vi "點檢.vi"() -> ()   [LabVIEW 2015]
uses:
  <vilib>/Utility/miscctls.llb/LVPointTypeDef.ctl
  <vilib>/userdefined/High Color/IMAQdx.ctl
panel:
  out "output cluster":T1
  in  "?":T2={"掃描速度"=1000, "功率"=80, "切割刀數"=10, "角度"=10.0, "掃描速度2"=1000, "功率2"=80, "切割刀數2"=10, "角度2"=10.0, "掃描速度3"=1000, "功率3"=80, "切割刀數3"=10, "角度3"=10.0, "掃描速度4"=1000, "功率4"=80, "切割刀數4"=10, "角度4"=10.0, "掃描速度5"=1000, "功率5"=80, "切割刀數5"=10, "左/右"=""} {"切割刀數5" min=0 max=10 step=1; "功率5" min=3 max=80 step=1; "掃描速度5" min=0 max=10000 step=10; "角度4" min=0.0 max=10.0 step=1.0; "角度3" min=0.0 max=10.0 step=1.0; "角度2" min=0.0 max=10.0 step=1.0; "角度" min=0.0 max=10.0 step=1.0; "切割刀數4" min=0 max=10 step=1; "功率4" min=3 max=80 step=1; "掃描速度4" min=0 max=1000 step=10; "切割刀數3" min=0 max=10 step=1; "功率3" min=3 max=80 step=1; "掃描速度3" min=0 max=1000 step=10; "切割刀數" min=0 max=10 step=1; "功率" min=3 max=80 step=1; "掃描速度" min=0 max=1000 step=10; "切割刀數2" max=10 step=1; "掃描速度2" min=0 max=1000 step=10; "功率2" min=3 max=80 step=1}
  in  "file (use dialog)":path=path "C:/Users/jyun.huang.MINAIK/Desktop/四穴雷切/參數設定/Data/參數設定"
  out "狀態：":string
  out "群組：":string
  out "帳號：":string
  in  "開啟檔案":bool
  in  "儲存檔案":bool
  in  "左/右":enum16{"オ", "右"}(ring)
  in  "雷射半徑":dbl min=0.0 max=220.0
  in  "雷射圓心座標":cluster{"X":dbl, "Y":dbl} {"X" min=0.0 max=220.0}
  in  "雷射觸發":bool
  in  "切割刀數":u32=2 min=2 max=85 step=1
  in  "掃描速率(刀速)":u16=220 max=2000 format="%0.0f"
  in  "功率":u8=70 max=80
  out "前後差異值":cluster{"X差":sgl, "Y差 ":sgl}
  in  "取像":bool
  in  "Tab Control":enum32{"原來圖片                      ", "後來圖片"}(tab)=enum."後來圖片"
  in  "找圓":bool
  in  "差值":bool
  out "原來圓心":cluster{"X ":sgl, "Y":sgl}
  in  "點檢":bool
  out "後來圓心":cluster{"X ":sgl, "Y":sgl}
  out "後來差值":cluster{"X差":sgl, "Y差 ":sgl}
  out "影像中心":cluster{"X":sgl, "Y":sgl}
  out "原來差值":cluster{"X差":sgl, "Y差 ":sgl}
  out "點檢 Action":T3
  out "Image":T4(plugin-control)
  in  "匯入圖片":bool
  in  "離開":bool
  # "每日點檢"
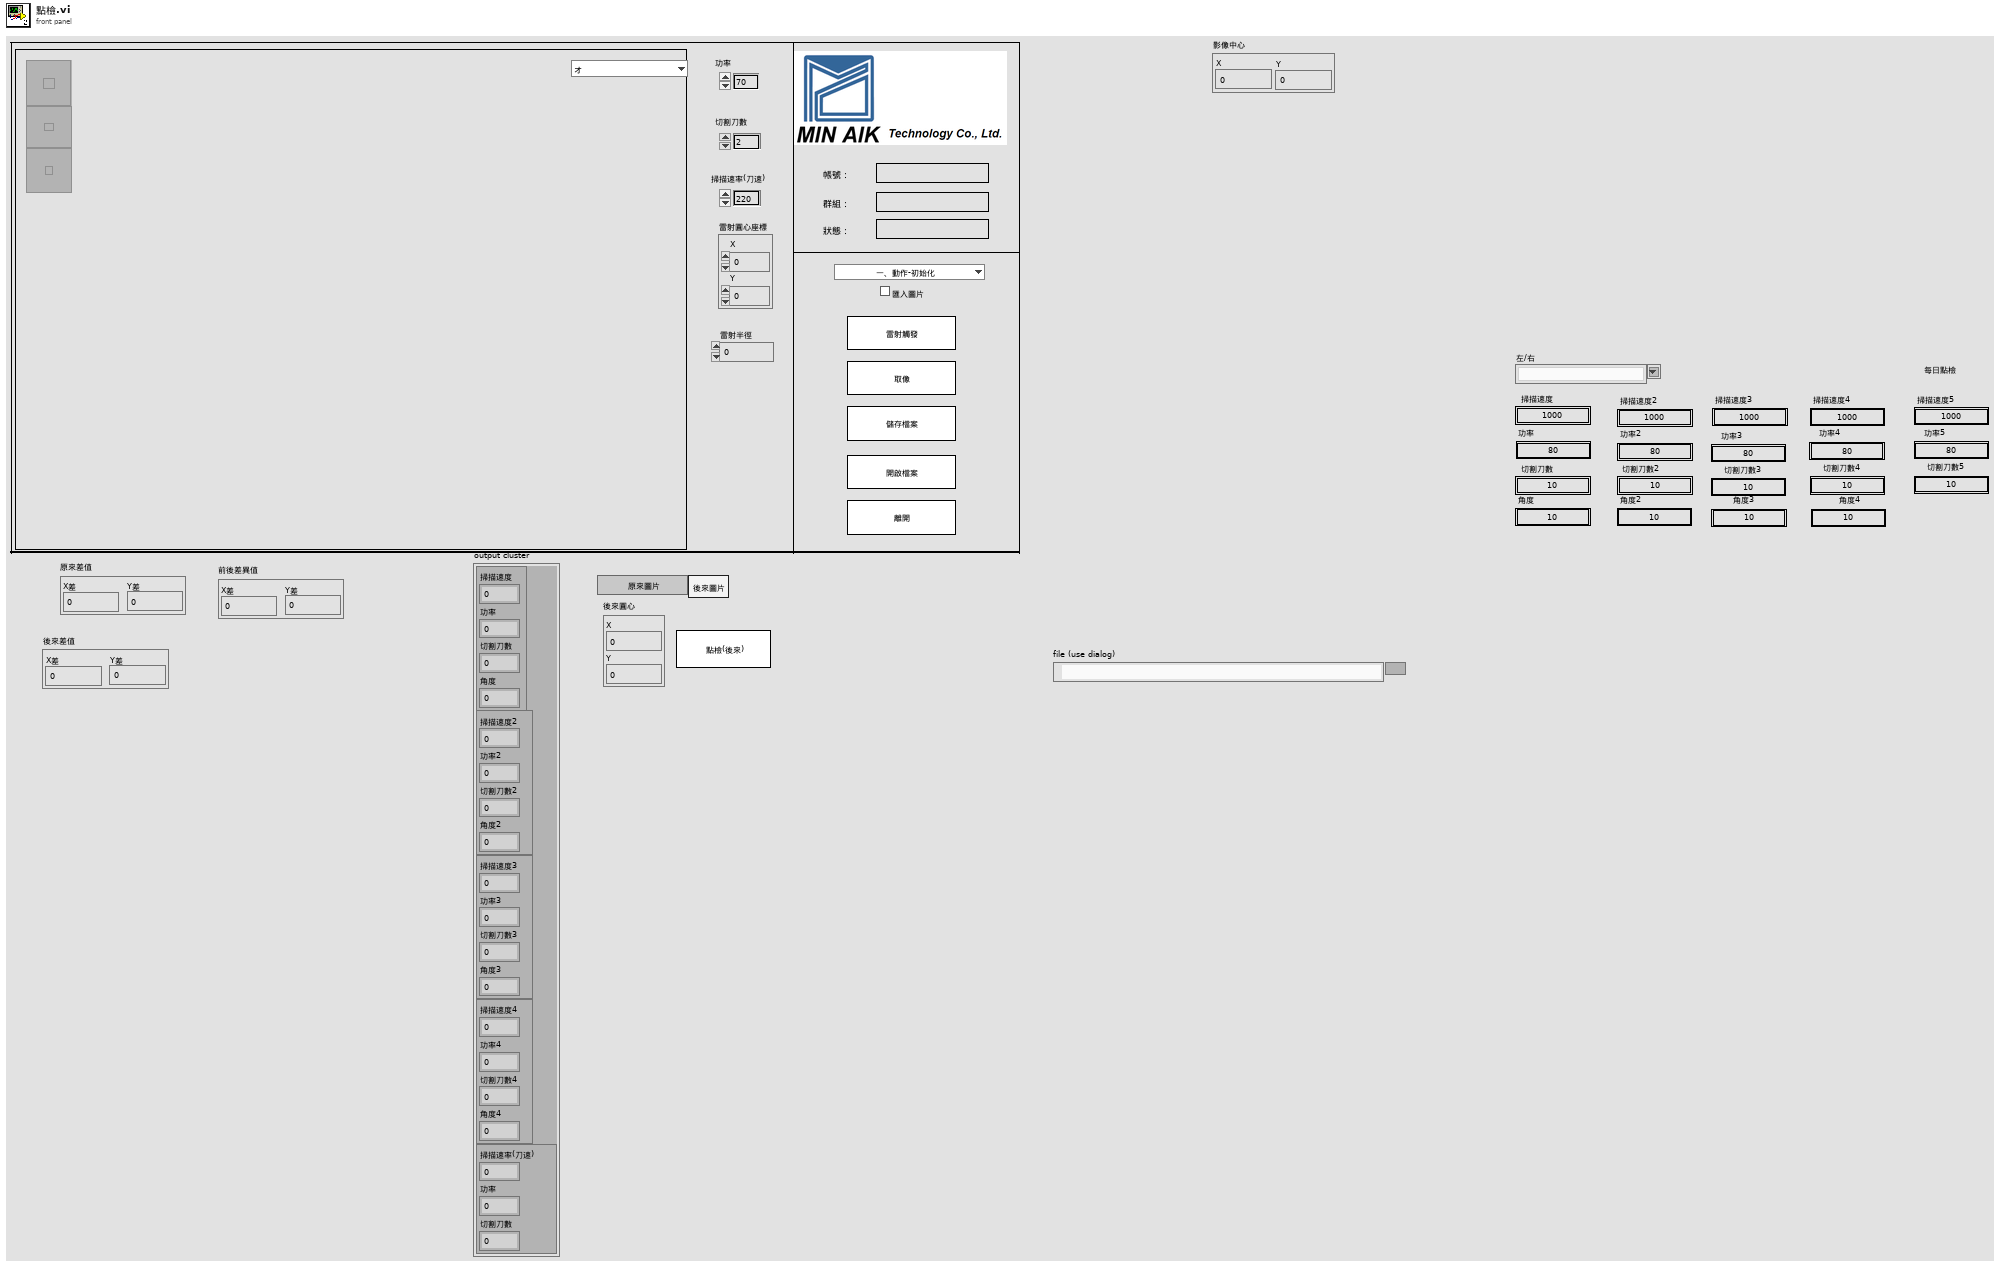
[diagram p1: front panel]
types:
  T1 = cluster{cluster{"掃描速度":i32, "功率":i32, "切割刀數":i32, "角度":dbl}, cluster{"掃描速度2":i32, "功率2":i32, "切割刀數2":i32, "角度2":dbl}, cluster{"掃描速度3":i32, "功率3":i32, "切割刀數3":i32, "角度3":dbl}, cluster{"掃描速度4":i32, "功率4":i32, "切割刀數4":i32, "角度4":dbl}, cluster{"掃描速率(刀速) ":u16, "功率":u8, "切割刀數":u32}}
  T2 = cluster{"掃描速度":i32, "功率":i32, "切割刀數":i32, "角度":dbl, "掃描速度2":i32, "功率2":i32, "切割刀數2":i32, "角度2":dbl, "掃描速度3":i32, "功率3":i32, "切割刀數3":i32, "角度3":dbl, "掃描速度4":i32, "功率4":i32, "切割刀數4":i32, "角度4":dbl, "掃描速度5":i32, "功率5":i32, "切割刀數5":i32, "左/右":string}
  T3 = typedef "點檢_Control_Main Action.ctl" = enum16{"一、動作-初始化", "二、動作-單次取像", "三、動作-測試", "四、動作-點檢", "五、動作-雷射寫入", "六、動作-雷射處發", "七、動作-離開", "1.0 功能-IO控制", "       1.1 IO-初始化", "       1.2 Set Point(EOT On)", "       1.3Set Point(EOT Off)", "       1.4Get Point(SOT)", "2.0功能-相機控制", "       2.1相機-初始化", "       2.2相機-取像", "       2.3相機-關閉", "3.0功能-影像控制", "       3.1影像-初始化", "       3.2影像-更新影像", "       3.3影像-儲存影像", "4.0功能-檢測", "       4.1檢測-初始化", "      4.2檢測-找圓(原來)", "      4.3檢測-找圓(後來)", "5.0功能-雷射控制", "      5.1雷射-初始化", "      5.2雷射-寫入數值", "      5.3雷射-讀出數值", "      5.4雷射-雷射觸發", "      5.5雷射-關閉", "6.0功能-檔案", "       6.1檔案-初始化", "       6.2檔案-儲存檔案", "       6.3檔案-開啟檔案", "       6.4檔案-匯入數值", "7.0 錯誤", "8.0等待", "       8.1等待(計算時間)", "9.0離開", "10.0功能-機台驗證", "      10.1機台驗證-測試", "      10.2機台驗證-檢測", "11.0對話視窗"}
  T4 = typedef "IMAQ Image.ctl" = refnum<image>
  T5 = typedef "LVPointTypeDef.ctl" = cluster{"Horizontal":i16, "Vertical":i16}
  T6 = typedef "IMAQdx.ctl" = refnum<k21>
  T7 = typedef "action_camera.ctl" = enum16{"初始化", "取像", "匯入影像", "結束"}
  T8 = typedef "Image action.ctl" = enum16{"初始化", "創造記憶體", "寫入圖片", "讀取圖片", "刪除圖片", "等待"}
  T9 = typedef "Action_Data.ctl" = enum16{"Initialize", "Get Data", "Set Data", "Delete Data", "Idle"}
  T10 = enum16{"RS232_Init ", "雷射準備訊號", "雷射觸發", "RS232_Close", "寫入雷射XY座標值與角度", "請求程式編號prog所有資訊", "開起導向光", "關閉導向光", "運行切換"}
  T11 = cluster{cluster{"掃描速度":i32, "功率":i32, "切割刀數":dbl, "左/右":string}, cluster{"掃描速度2":i32, "功率2":i32, "切割刀數2":dbl, "左/右":string}, cluster{"掃描速度3":i32, "功率3":i32, "切割刀數3":dbl, "左/右":string}, cluster{"掃描速度4":i32, "功率4":i32, "切割刀數4":dbl, "左/右":string}, cluster{"掃描速度5":i32, "功率5":i32, "切割刀數5":dbl, "左/右":string}}
  T12 = cluster{"功率":u8, "掃描速率(刀速) ":u16, "雷射半徑":dbl, "刀數":u32}
  T13 = cluster{"ROI":cluster{"Global Rectangle":i32[], "Contours":cluster{"Contour Type":u32, "ROI Type":u32, "Points":i32[]}[]}, "圓心 (Pixels)":cluster{"X":sgl, "Y":sgl}}
  T14 = typedef "Image Type" = u32
  T15 = cluster{"Global Rectangle":i32[], "Contours":cluster{"Contour Type":u32, "ROI Type":u32, "Points":i32[]}[]}
  T16 = cluster{"功率":u8, "掃描速率(刀速) ":u16, "雷射半徑":dbl, "切割刀數":u32}
  T17 = cluster{"掃描速度5":i32, "功率5":i32, "切割刀數5":dbl, "左/右":string}
  T18 = cluster{"掃描速度4":i32, "功率4":i32, "切割刀數4":i32, "角度4":dbl}
  T19 = cluster{"掃描速度2":i32, "功率2":i32, "切割刀數2":i32, "角度2":dbl}
  T20 = cluster{"掃描速度3":i32, "功率3":i32, "切割刀數3":i32, "角度3":dbl}
  T21 = cluster{"掃描速度":i32, "功率":i32, "切割刀數":i32, "角度":dbl}
  T22 = cluster{"name or relative path":string, "Variant":variant}
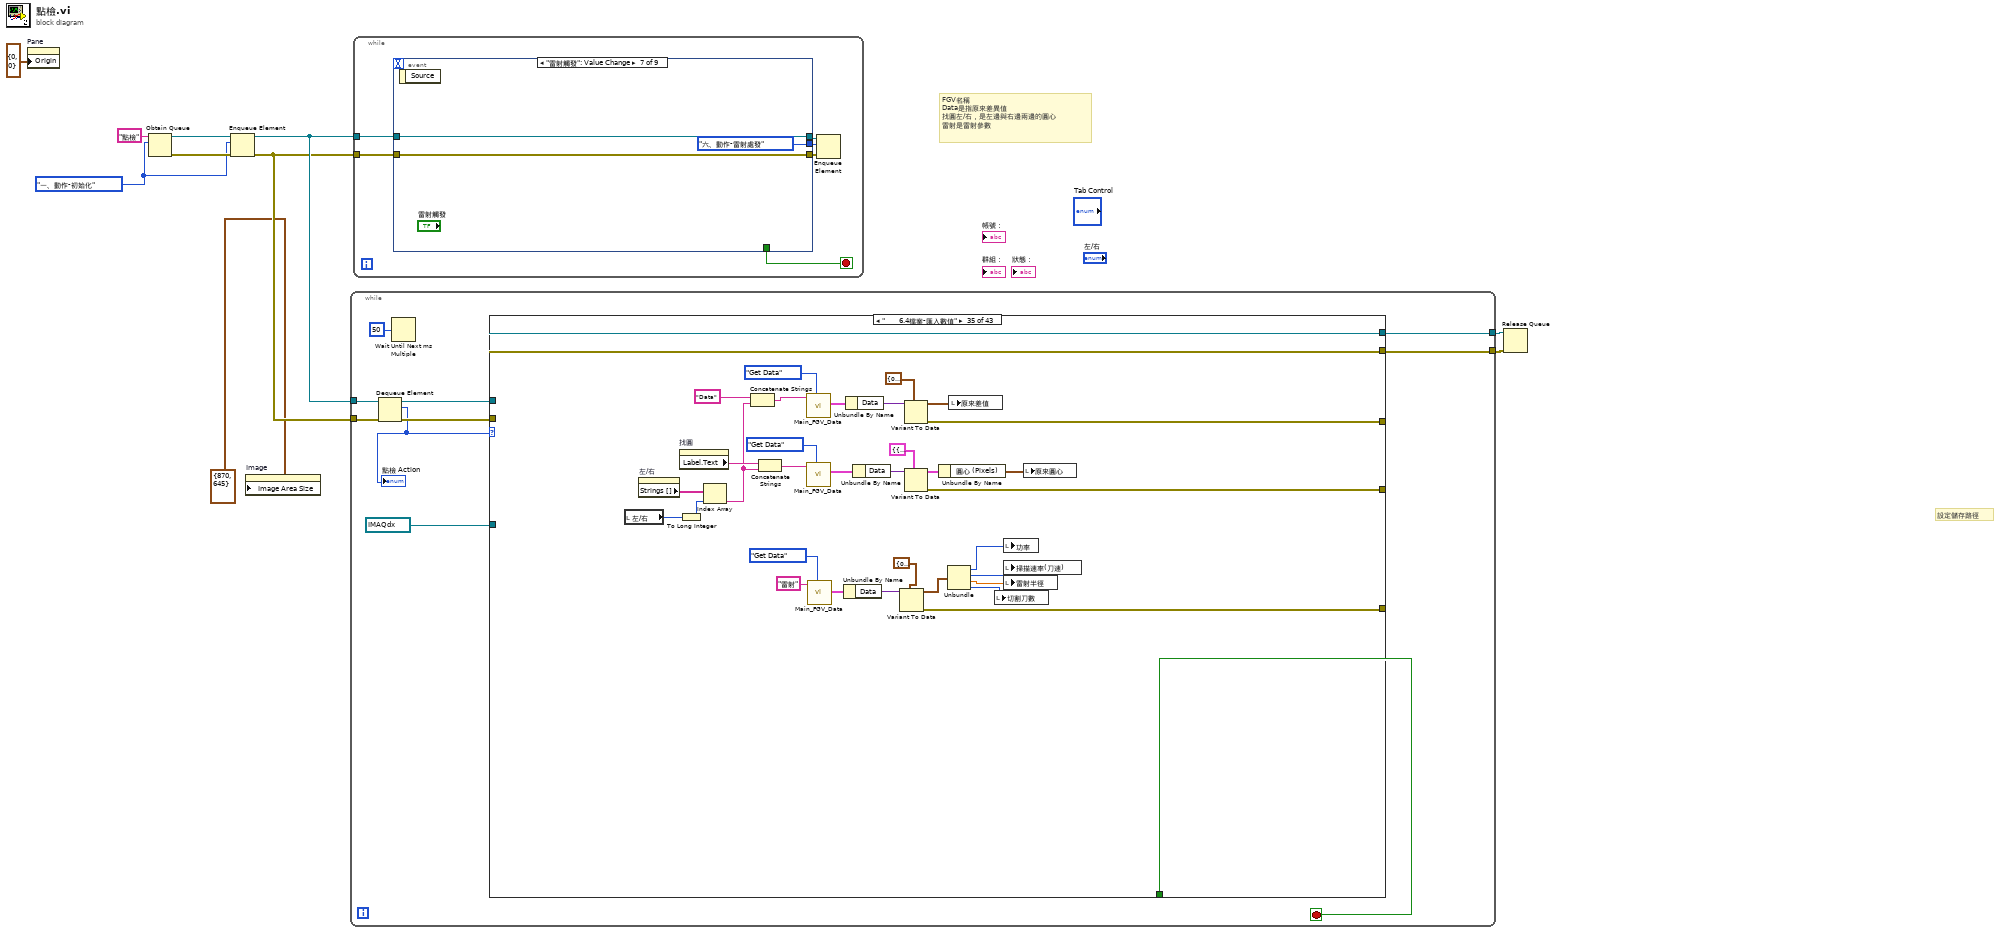
[diagram p0: block diagram]
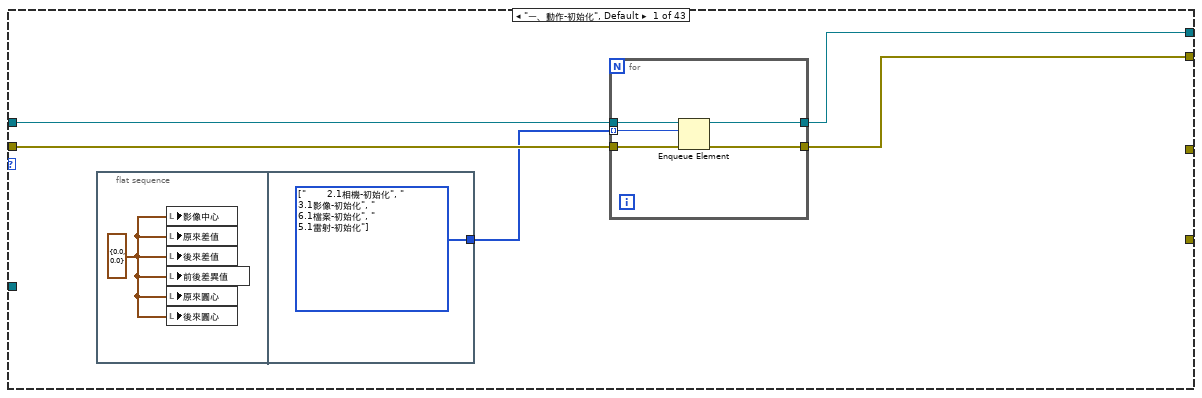
[diagram p2: hidden frame]
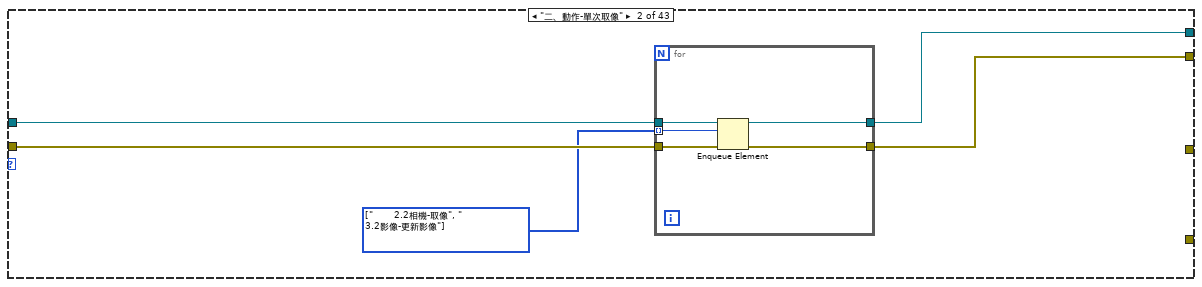
[diagram p3: hidden frame]
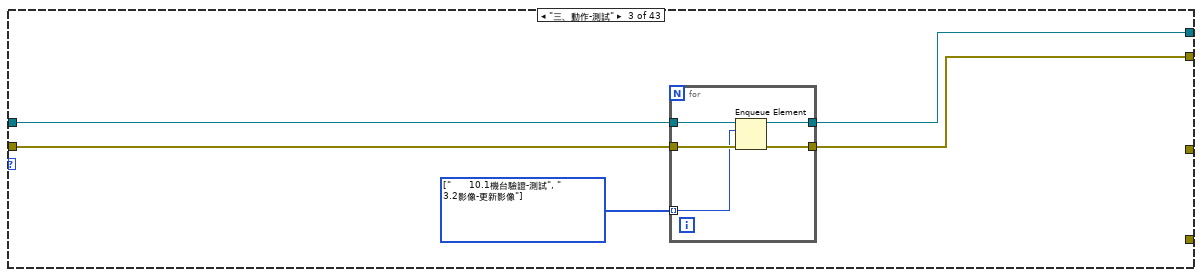
[diagram p4: hidden frame]
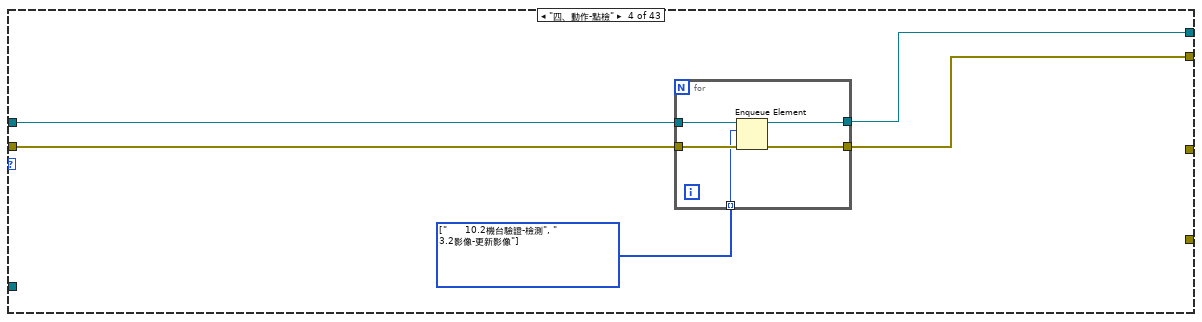
[diagram p5: hidden frame]
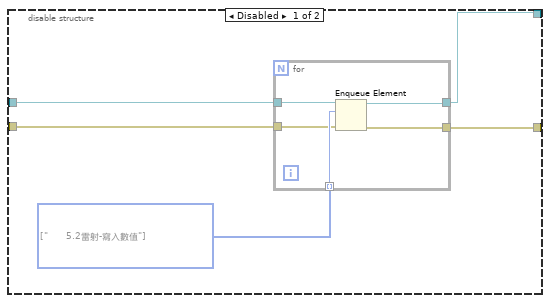
[diagram p7: hidden frame]
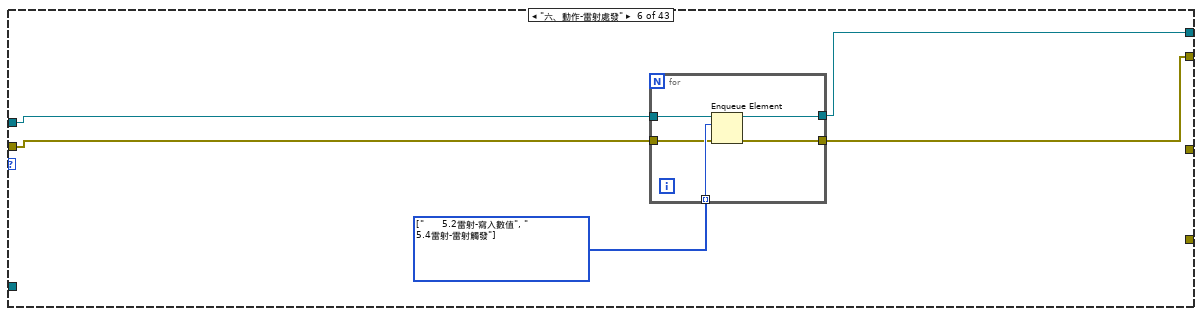
[diagram p8: hidden frame]
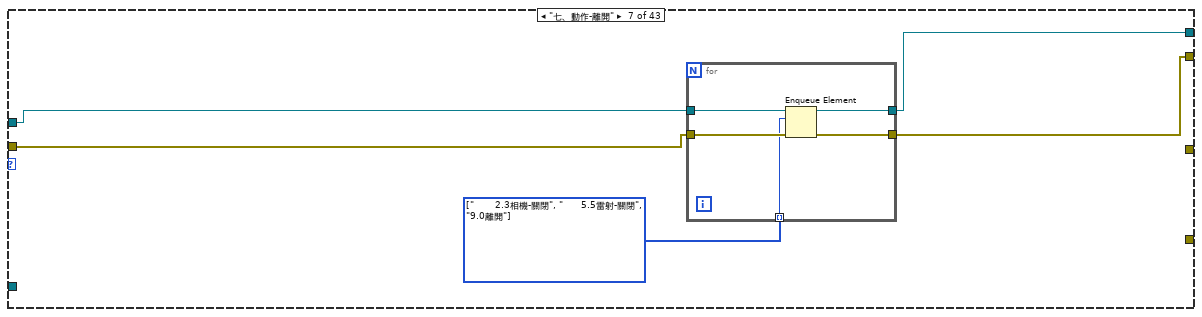
[diagram p9: hidden frame]
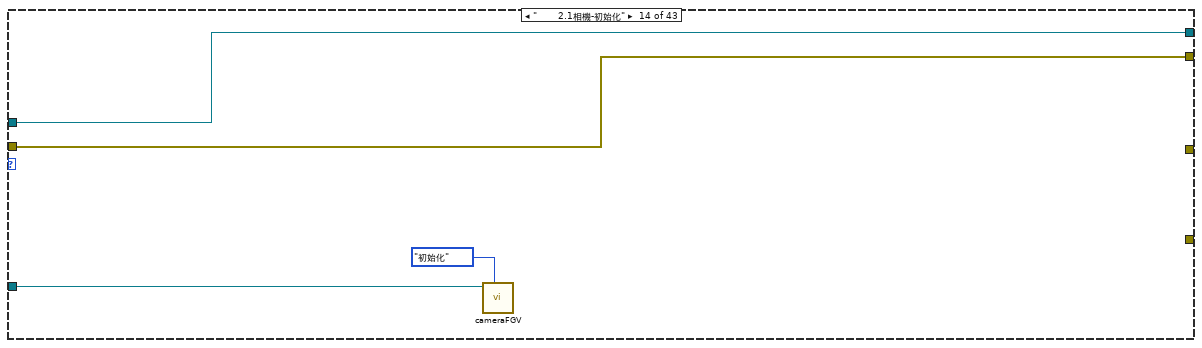
[diagram p16: hidden frame]
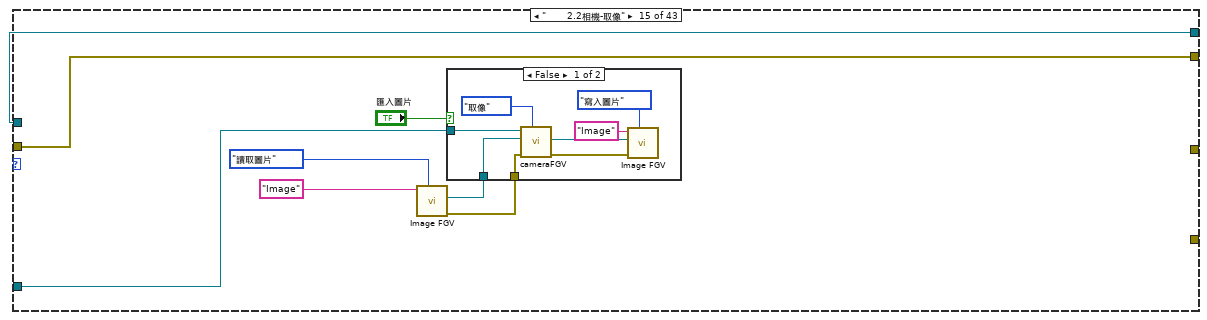
[diagram p17: hidden frame]
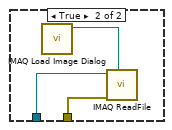
[diagram p18: hidden frame]
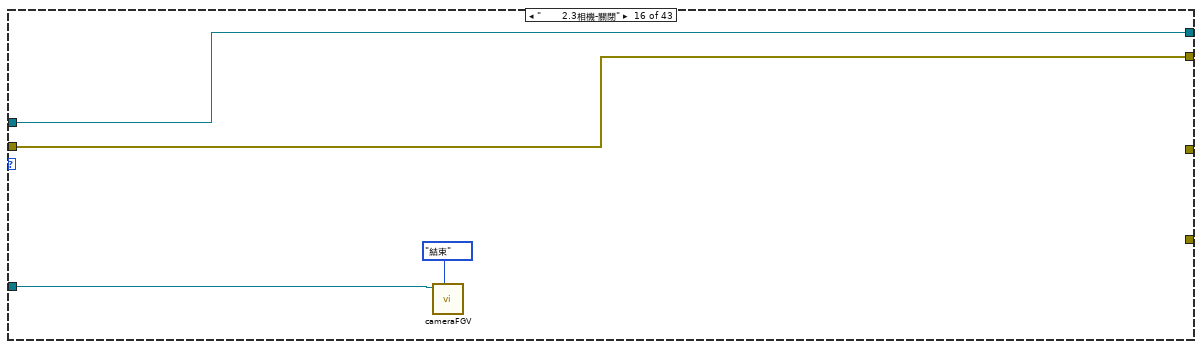
[diagram p19: hidden frame]
diagram:
  w3 = 點檢_Control_Main_Action."一、動作-初始化" ("點檢 Action")
  # "FGV名稱\nData是指原來差異值\n找圓左/右，是左邊與右邊兩邊的圓心\n雷射是雷射參數"
  # "設定儲存路徑"
  n1 = property on="Pane" class="Pane"("Origin"=T5 {"Horizontal"=0, "Vertical"=0}) -> ()  [unwired: 2 in, 2 out]
  n2 = Obtain Queue(name (unnamed)="點檢", element data type=w3) -> (queue out=w9:refnum<queue>, error out=w8:errorcluster)  [unwired: 3 in, 1 out]
  n3 = Enqueue Element(queue=w9, element=w3, error in (no error)=w8) -> (queue out=w7:refnum<queue>, error out=w6:errorcluster)  [unwired: 1 in, 1 out]
  n4 = property on="Image" class="ImageControl"("Image Area Size"=cluster{"Width":u32, "Height":u32} {"Width"=870, "Height"=645} ("Image Area:Size:All Elements")) -> ()  [unwired: 2 in, 2 out]
  n5 = while {
    tunnel: w7 -> [w20]
    tunnel: w6 -> [w19]
    tunnel: [w15] -> w5
    tunnel: [w14] -> w4
    stop <- w18 stop-if-true
    n6 = Dequeue Element(queue=w20, error in (no error)=w19) -> (queue out=w17:refnum<queue>, element=w11:T3, error out=w16:errorcluster)  [unwired: 1 in, 1 out]
    "點檢 Action" <- w11
    n7 = Wait Until Next ms Multiple(millisecond multiple=u32 50) -> ()  [unwired: 1 out]
    n8 = case shown="\"       6.4檔案-匯入數值\"" w11 {
      tunnel: [_ _ _ _ _ _ _ _ _ _ _ _ _ _ _ _ _ _ _ _ _ _ _ _ _ _ _ _ _ _ _ _ _ _ _ _ _ _ TRUE _ _ _ _] -> w18
      tunnel: w17 -> [w22 w37 w47 w57 w66 w82 w92 w100 w102 w104 w106 w108 w110 w113 w117 w134 w139 w143 w158 w160 w162 w164 w180 w186 w188 w193 w217 w270 w273 w285 w287 w290 w304 w353 w396 w398 w400 w402 w404 w407 w441 w472 w474]
      tunnel: w16 -> [w25 w36 w46 w56 w65 w81 w91 w99 w101 w103 w105 w107 w109 w111 w116 w137 w138 w140 w154 w159 w161 w163 w179 w185 w187 w192 w216 w269 w272 w284 w286 w289 w303 w352 w395 w397 w399 w401 w403 w406 w440 w471 w473]
      tunnel: [w23 w35 w45 w55 w64 w80 w90 w100 w102 w104 w106 w108 w110 w113 w117 w134 w139 w143 w158 w160 w162 w164 w178 w186 w188 w193 w217 w270 w273 w285 w287 w290 w304 w354 w396 w398 w400 w402 w404 w407 w441 w472 w474] -> w15
      tunnel: [w24 w34 w44 w54 w63 w79 w89 w99 w101 w103 w105 w107 w109 w111 w116 w137 w138 w140 w154 w159 w161 w163 w177 w185 w187 w192 w216 w269 w272 w284 w286 w289 w303 w351 w395 w397 w399 w401 w403 w406 w440 w471 w473] -> w14
      tunnel: T6 "cam0" ("Session In") -> [_ _ _ _ _ _ _ _ _ _ _ _ _ w112 w118 w136 _ _ _ _ _ _ _ _ _ _ _ _ _ _ _ _ _ _ _ _ _ _ _ _ _ _ _]
      tunnel: [_ _ _ _ _ _ _ _ _ _ _ _ _ _ _ _ _ _ _ _ _ _ _ _ _ _ _ _ _ _ _ _ _ w349 w375 _ _ _ _ _ _ _ _] -> _
      tunnel: [_ _ _ _ _ _ _ _ _ _ _ _ _ _ _ _ _ _ _ _ _ _ _ _ _ _ _ _ _ _ _ _ _ w348 w374 _ _ _ _ _ _ _ _] -> _
      tunnel: [_ _ _ _ _ _ _ _ _ _ _ _ _ _ _ _ _ _ _ _ _ _ _ _ _ _ _ _ _ _ _ _ _ _ w367 _ _ _ _ _ _ _ _] -> _
      frame "一、動作-初始化", Default {
        n9 = flat-sequence {
          tunnel: [w27] -> w21
          frame #0 {
            w26 = cluster{"X":sgl, "Y":sgl} {"X"=0.0, "Y"=0.0} ("影像中心")
            n10 = local write "影像中心"(w26) -> ()
            n11 = local write "原來差值"(w26) -> ()
            n12 = local write "後來差值"(w26) -> ()
            n13 = local write "前後差異值"(w26) -> ()
            n14 = local write "原來圓心"(w26) -> ()
            n15 = local write "後來圓心"(w26) -> ()
          }
          frame #1 {
            w27 = T3[] [enum."       2.1相機-初始化", enum."       3.1影像-初始化", enum."       6.1檔案-初始化", enum."      5.1雷射-初始化"] items=["一、動作-初始化", "二、動作-單次取像", "三、動作-測試", "四、動作-點檢", "五、動作-雷射寫入", "六、動作-雷射處發", "七、動作-離開", "1.0 功能-IO控制", "       1.1 IO-初始化", "       1.2 Set Point(EOT On)", "       1.3Set Point(EOT Off)", "       1.4Get Point(SOT)", "2.0功能-相機控制", "       2.1相機-初始化", "       2.2相機-取像", "       2.3相機-關閉", "3.0功能-影像控制", "       3.1影像-初始化", "       3.2影像-更新影像", "       3.3影像-儲存影像", "4.0功能-檢測", "       4.1檢測-初始化", "      4.2檢測-找圓(原來)", "      4.3檢測-找圓(後來)", "5.0功能-雷射控制", "      5.1雷射-初始化", "      5.2雷射-寫入數值", "      5.3雷射-讀出數值", "      5.4雷射-雷射觸發", "      5.5雷射-關閉", "6.0功能-檔案", "       6.1檔案-初始化", "       6.2檔案-儲存檔案", "       6.3檔案-開啟檔案", "       6.4檔案-匯入數值", "7.0 錯誤", "8.0等待", "       8.1等待(計算時間)", "9.0離開", "10.0功能-機台驗證", "      10.1機台驗證-測試", "      10.2機台驗證-檢測", "11.0對話視窗"]
          }
        }
        n16 = for {
          tunnel: w22 -> [w32]
          tunnel: w25 -> [w31]
          tunnel: [w30] -> w24
          tunnel: [w29] -> w23
          tunnel: w21 -> [w28] mode=indexing
          n17 = Enqueue Element(queue=w32, element=w28, error in (no error)=w31) -> (queue out=w29:refnum<queue>, error out=w30:errorcluster)  [unwired: 1 in, 1 out]
        }
      }
      frame "二、動作-單次取像" {
        w33 = T3[] [enum."       2.2相機-取像", enum."       3.2影像-更新影像"] items=["一、動作-初始化", "二、動作-單次取像", "三、動作-測試", "四、動作-點檢", "五、動作-雷射寫入", "六、動作-雷射處發", "七、動作-離開", "1.0 功能-IO控制", "       1.1 IO-初始化", "       1.2 Set Point(EOT On)", "       1.3Set Point(EOT Off)", "       1.4Get Point(SOT)", "2.0功能-相機控制", "       2.1相機-初始化", "       2.2相機-取像", "       2.3相機-關閉", "3.0功能-影像控制", "       3.1影像-初始化", "       3.2影像-更新影像", "       3.3影像-儲存影像", "4.0功能-檢測", "       4.1檢測-初始化", "      4.2檢測-找圓(原來)", "      4.3檢測-找圓(後來)", "5.0功能-雷射控制", "      5.1雷射-初始化", "      5.2雷射-寫入數值", "      5.3雷射-讀出數值", "      5.4雷射-雷射觸發", "      5.5雷射-關閉", "6.0功能-檔案", "       6.1檔案-初始化", "       6.2檔案-儲存檔案", "       6.3檔案-開啟檔案", "       6.4檔案-匯入數值", "7.0 錯誤", "8.0等待", "       8.1等待(計算時間)", "9.0離開", "10.0功能-機台驗證", "      10.1機台驗證-測試", "      10.2機台驗證-檢測", "11.0對話視窗"]
        n18 = for {
          tunnel: w37 -> [w42]
          tunnel: w36 -> [w41]
          tunnel: [w40] -> w35
          tunnel: [w39] -> w34
          tunnel: w33 -> [w38] mode=indexing
          n19 = Enqueue Element(queue=w42, element=w38, error in (no error)=w41) -> (queue out=w40:refnum<queue>, error out=w39:errorcluster)  [unwired: 1 in, 1 out]
        }
      }
      frame "三、動作-測試" {
        w43 = T3[] [enum."      10.1機台驗證-測試", enum."       3.2影像-更新影像"] items=["一、動作-初始化", "二、動作-單次取像", "三、動作-測試", "四、動作-點檢", "五、動作-雷射寫入", "六、動作-雷射處發", "七、動作-離開", "1.0 功能-IO控制", "       1.1 IO-初始化", "       1.2 Set Point(EOT On)", "       1.3Set Point(EOT Off)", "       1.4Get Point(SOT)", "2.0功能-相機控制", "       2.1相機-初始化", "       2.2相機-取像", "       2.3相機-關閉", "3.0功能-影像控制", "       3.1影像-初始化", "       3.2影像-更新影像", "       3.3影像-儲存影像", "4.0功能-檢測", "       4.1檢測-初始化", "      4.2檢測-找圓(原來)", "      4.3檢測-找圓(後來)", "5.0功能-雷射控制", "      5.1雷射-初始化", "      5.2雷射-寫入數值", "      5.3雷射-讀出數值", "      5.4雷射-雷射觸發", "      5.5雷射-關閉", "6.0功能-檔案", "       6.1檔案-初始化", "       6.2檔案-儲存檔案", "       6.3檔案-開啟檔案", "       6.4檔案-匯入數值", "7.0 錯誤", "8.0等待", "       8.1等待(計算時間)", "9.0離開", "10.0功能-機台驗證", "      10.1機台驗證-測試", "      10.2機台驗證-檢測", "11.0對話視窗"]
        n20 = for {
          tunnel: w47 -> [w52]
          tunnel: w46 -> [w51]
          tunnel: [w50] -> w45
          tunnel: [w49] -> w44
          tunnel: w43 -> [w48] mode=indexing
          n21 = Enqueue Element(queue=w52, element=w48, error in (no error)=w51) -> (queue out=w50:refnum<queue>, error out=w49:errorcluster)  [unwired: 1 in, 1 out]
        }
      }
      frame "四、動作-點檢" {
        w53 = T3[] [enum."      10.2機台驗證-檢測", enum."       3.2影像-更新影像"] items=["一、動作-初始化", "二、動作-單次取像", "三、動作-測試", "四、動作-點檢", "五、動作-雷射寫入", "六、動作-雷射處發", "七、動作-離開", "1.0 功能-IO控制", "       1.1 IO-初始化", "       1.2 Set Point(EOT On)", "       1.3Set Point(EOT Off)", "       1.4Get Point(SOT)", "2.0功能-相機控制", "       2.1相機-初始化", "       2.2相機-取像", "       2.3相機-關閉", "3.0功能-影像控制", "       3.1影像-初始化", "       3.2影像-更新影像", "       3.3影像-儲存影像", "4.0功能-檢測", "       4.1檢測-初始化", "      4.2檢測-找圓(原來)", "      4.3檢測-找圓(後來)", "5.0功能-雷射控制", "      5.1雷射-初始化", "      5.2雷射-寫入數值", "      5.3雷射-讀出數值", "      5.4雷射-雷射觸發", "      5.5雷射-關閉", "6.0功能-檔案", "       6.1檔案-初始化", "       6.2檔案-儲存檔案", "       6.3檔案-開啟檔案", "       6.4檔案-匯入數值", "7.0 錯誤", "8.0等待", "       8.1等待(計算時間)", "9.0離開", "10.0功能-機台驗證", "      10.1機台驗證-測試", "      10.2機台驗證-檢測", "11.0對話視窗"]
        n22 = for {
          tunnel: w57 -> [w62]
          tunnel: w56 -> [w61]
          tunnel: [w60] -> w55
          tunnel: [w59] -> w54
          tunnel: w53 -> [w58] mode=indexing
          n23 = Enqueue Element(queue=w62, element=w58, error in (no error)=w61) -> (queue out=w60:refnum<queue>, error out=w59:errorcluster)  [unwired: 1 in, 1 out]
        }
      }
      frame "五、動作-雷射寫入" {
        n24 = disable-structure shown="Enabled" {
          disable-tunnel: w66 -> [w70 w77]
          disable-tunnel: w65 -> [w69 w78]
          disable-tunnel: [w68 w77] -> w64
          disable-tunnel: [w67 w78] -> w63
          frame Disabled {
            w71 = T3[] [enum."      5.2雷射-寫入數值"] items=["一、動作-初始化", "二、動作-單次取像", "三、動作-測試", "四、動作-點檢", "五、動作-雷射寫入", "六、動作-雷射處發", "七、動作-離開", "1.0 功能-IO控制", "       1.1 IO-初始化", "       1.2 Set Point(EOT On)", "       1.3Set Point(EOT Off)", "       1.4Get Point(SOT)", "2.0功能-相機控制", "       2.1相機-初始化", "       2.2相機-取像", "       2.3相機-關閉", "3.0功能-影像控制", "       3.1影像-初始化", "       3.2影像-更新影像", "       3.3影像-儲存影像", "4.0功能-檢測", "       4.1檢測-初始化", "      4.2檢測-找圓(原來)", "      4.3檢測-找圓(後來)", "5.0功能-雷射控制", "      5.1雷射-初始化", "      5.2雷射-寫入數值", "      5.3雷射-讀出數值", "      5.4雷射-雷射觸發", "      5.5雷射-關閉", "6.0功能-檔案", "       6.1檔案-初始化", "       6.2檔案-儲存檔案", "       6.3檔案-開啟檔案", "       6.4檔案-匯入數值", "7.0 錯誤", "8.0等待", "       8.1等待(計算時間)", "9.0離開", "10.0功能-機台驗證", "      10.1機台驗證-測試", "      10.2機台驗證-檢測", "11.0對話視窗"]
            n25 = for {
              tunnel: [w76] -> w68
              tunnel: [w75] -> w67
              tunnel: w71 -> [w74] mode=indexing
              tunnel: w70 -> [w73]
              tunnel: w69 -> [w72]
              n26 = Enqueue Element(queue=w73, element=w74, error in (no error)=w72) -> (queue out=w76:refnum<queue>, error out=w75:errorcluster)  [unwired: 1 in, 1 out]
            }
          }
          frame Enabled {
          }
        }
      }
      frame "六、動作-雷射處發" {
        w83 = T3[] [enum."      5.2雷射-寫入數值", enum."      5.4雷射-雷射觸發"] items=["一、動作-初始化", "二、動作-單次取像", "三、動作-測試", "四、動作-點檢", "五、動作-雷射寫入", "六、動作-雷射處發", "七、動作-離開", "1.0 功能-IO控制", "       1.1 IO-初始化", "       1.2 Set Point(EOT On)", "       1.3Set Point(EOT Off)", "       1.4Get Point(SOT)", "2.0功能-相機控制", "       2.1相機-初始化", "       2.2相機-取像", "       2.3相機-關閉", "3.0功能-影像控制", "       3.1影像-初始化", "       3.2影像-更新影像", "       3.3影像-儲存影像", "4.0功能-檢測", "       4.1檢測-初始化", "      4.2檢測-找圓(原來)", "      4.3檢測-找圓(後來)", "5.0功能-雷射控制", "      5.1雷射-初始化", "      5.2雷射-寫入數值", "      5.3雷射-讀出數值", "      5.4雷射-雷射觸發", "      5.5雷射-關閉", "6.0功能-檔案", "       6.1檔案-初始化", "       6.2檔案-儲存檔案", "       6.3檔案-開啟檔案", "       6.4檔案-匯入數值", "7.0 錯誤", "8.0等待", "       8.1等待(計算時間)", "9.0離開", "10.0功能-機台驗證", "      10.1機台驗證-測試", "      10.2機台驗證-檢測", "11.0對話視窗"]
        n27 = for {
          tunnel: [w88] -> w80
          tunnel: [w87] -> w79
          tunnel: w83 -> [w86] mode=indexing
          tunnel: w82 -> [w85]
          tunnel: w81 -> [w84]
          n28 = Enqueue Element(queue=w85, element=w86, error in (no error)=w84) -> (queue out=w88:refnum<queue>, error out=w87:errorcluster)  [unwired: 1 in, 1 out]
        }
      }
      frame "七、動作-離開" {
        w93 = T3[] [enum."       2.3相機-關閉", enum."      5.5雷射-關閉", enum."9.0離開"] items=["一、動作-初始化", "二、動作-單次取像", "三、動作-測試", "四、動作-點檢", "五、動作-雷射寫入", "六、動作-雷射處發", "七、動作-離開", "1.0 功能-IO控制", "       1.1 IO-初始化", "       1.2 Set Point(EOT On)", "       1.3Set Point(EOT Off)", "       1.4Get Point(SOT)", "2.0功能-相機控制", "       2.1相機-初始化", "       2.2相機-取像", "       2.3相機-關閉", "3.0功能-影像控制", "       3.1影像-初始化", "       3.2影像-更新影像", "       3.3影像-儲存影像", "4.0功能-檢測", "       4.1檢測-初始化", "      4.2檢測-找圓(原來)", "      4.3檢測-找圓(後來)", "5.0功能-雷射控制", "      5.1雷射-初始化", "      5.2雷射-寫入數值", "      5.3雷射-讀出數值", "      5.4雷射-雷射觸發", "      5.5雷射-關閉", "6.0功能-檔案", "       6.1檔案-初始化", "       6.2檔案-儲存檔案", "       6.3檔案-開啟檔案", "       6.4檔案-匯入數值", "7.0 錯誤", "8.0等待", "       8.1等待(計算時間)", "9.0離開", "10.0功能-機台驗證", "      10.1機台驗證-測試", "      10.2機台驗證-檢測", "11.0對話視窗"]
        n29 = for {
          tunnel: w92 -> [w98]
          tunnel: w91 -> [w97]
          tunnel: [w96] -> w90
          tunnel: [w95] -> w89
          tunnel: w93 -> [w94] mode=indexing
          n30 = Enqueue Element(queue=w98, element=w94, error in (no error)=w97) -> (queue out=w96:refnum<queue>, error out=w95:errorcluster)  [unwired: 1 in, 1 out]
        }
      }
      frame "1.0 功能-IO控制" {
      }
      frame "       1.1 IO-初始化" {
      }
      frame "       1.2 Set Point(EOT On)" {
      }
      frame "       1.3Set Point(EOT Off)" {
      }
      frame "       1.4Get Point(SOT)" {
      }
      frame "2.0功能-相機控制" {
      }
      frame "       2.1相機-初始化" {
        n31 = call "cameraFGV.vi"("action_camera"=action_camera."初始化", "Session In"=w112) -> ()  [unwired: 7 in, 3 out]
      }
      frame "       2.2相機-取像" {
        n32 = call "Image FGV.vi"("Image action"=Image_action."讀取圖片", "圖片名稱"="Image") -> ("error out"=w119:errorcluster, "Image Out"=w120:T4)  [unwired: 8 in]
        n33 = case shown="False" "匯入圖片" {
          tunnel: w120 -> [w130 w133]
          tunnel: w119 -> [w129 w132]
          tunnel: w118 -> [w128 _]
          frame False {
            n34 = call "cameraFGV.vi"("action_camera"=action_camera."取像", "error constant"=w129, "Image In"=w130, "Session In"=w128) -> ("error constant 2"=w127:errorcluster, "Image Out"=w126:T4)  [unwired: 5 in, 1 out]
            n35 = call "Image FGV.vi"("Image action"=Image_action."寫入圖片", "error in (no error)"=w127, "Image In"=w126, "圖片名稱"="Image") -> ()  [unwired: 6 in, 2 out]
          }
          frame True {
            n36 = call "IMAQ Load Image Dialog"() -> ("Path"=w131:path)  [unwired: 9 in, 2 out]
            n37 = call "IMAQ ReadFile"("File Path"=w131, "error in (no error)"=w132, "Image"=w133) -> ()  [unwired: 4 in, 5 out]
          }
        }
      }
      frame "       2.3相機-關閉" {
        n38 = call "cameraFGV.vi"("action_camera"=action_camera."結束", "Session In"=w136) -> ()  [unwired: 7 in, 3 out]
      }
      frame "3.0功能-影像控制" {
      }
      frame "       3.1影像-初始化" {
        w141 = T14[] [0] items=["Grayscale (U8)", "Grayscale (I16)", "Grayscale (SGL)", "Complex (CSG)", "RGB (U32)", "HSL (U32)", "RGB (U64)", "Grayscale (U16)"]
        n39 = call "Image FGV.vi"("Image action"=Image_action."初始化") -> ("error out"=w144:errorcluster)  [unwired: 9 in, 1 out]
        n40 = for {
          tunnel: w144 -> [w149]
          tunnel: string[] ["Image"] -> [w147] mode=indexing
          tunnel: w141 -> [w146] mode=indexing
          n41 = call "Image FGV.vi"("Image action"=Image_action."創造記憶體", "error in (no error)"=w149, "Image Type"=w146, "圖片名稱"=w147) -> ()  [unwired: 6 in, 2 out]
        }
      }
      frame "       3.2影像-更新影像" {
        n42 = call "Image FGV.vi"("Image action"=Image_action."讀取圖片", "圖片名稱"="Image") -> ("error out"=w153:errorcluster, "Image Out"=w152:T4)  [unwired: 8 in]
        n43 = property on="Image" class="ImageControl"("Zoom to Fit Mode"=TRUE) -> ()  [unwired: 2 in, 2 out]
        n44 = call "點檢_VI_畫十字線.vi"("error in (no error)"=w153, "Refnum in"=w152) -> ("中心點"=→"影像中心":cluster{sgl, sgl}, "Refnum out"=→"Image":T4)  [unwired: 7 in, 1 out]
      }
      frame "       3.3影像-儲存影像" {
      }
      frame "4.0功能-檢測" {
      }
      frame "       4.1檢測-初始化" {
      }
      frame "      4.2檢測-找圓(原來)" {
        n45 = call "Image FGV.vi"("Image action"=Image_action."讀取圖片", "圖片名稱"="Image") -> ("Image Out"=w182:T4)  [unwired: 8 in, 1 out]
        n46 = property on="Image" class="ImageControl"() -> ("ROI"=w174:T15)  [unwired: 2 in, 2 out]
        n47 = local read "左/右"() -> (w169:enum16{"オ", "右"})
        n48 = call "點檢_VI_找圓.vi"("ROI Descriptor"=w174, "Image"=w182) -> ("圓心 (Pixels)"=w172:cluster{"X":sgl, "Y":sgl})  [unwired: 6 in, 3 out]
        "原來圓心" <- w172
        n49 = property on="左/右" class="Enum (strict)"() -> ("Strings []"=w171:string[])  [unwired: 2 in, 2 out]
        n50 = property on="找圓" class="Bool"() -> ("Label.Text"=w168:string)  [unwired: 2 in, 2 out]
        n51 = Bundle("ROI"=w174, "圓心 (Pixels)"=w172) -> (w173:T13)  [unwired: 1 in]
        n52 = To Long Integer(number=w169) -> (32bit integer=w170:i32)
        n53 = Index Array(array=w171, index=w170) -> (element=w167:string)
        n54 = To Variant(anything=w173) -> (Variant=w175:variant)
        n55 = Concatenate Strings(w168, w167) -> (w165:string)
        n56 = Bundle(w165, "Variant"=w175) -> (w166:cluster{string, "Variant":variant})  [unwired: 1 in]
        n57 = call "Main_FGV_Data.vi"("Action_Data"=Action_Data."Set Data", "Data In"=w166, "Data name"=w165) -> ()  [unwired: 7 in, 2 out]
        n58 = Enqueue Element(queue=w180, element=點檢_Control_Main_Action."       3.2影像-更新影像", error in (no error)=w179) -> (queue out=w178:refnum<queue>, error out=w177:errorcluster)  [unwired: 1 in, 1 out]
      }
      frame "      4.3檢測-找圓(後來)" {
      }
      frame "5.0功能-雷射控制" {
      }
      frame "      5.1雷射-初始化" {
        n59 = call "RS232 Device.vi"() -> ("error out"=w189:errorcluster, "COM"=w190:refnum<visa-resource-name>)  [unwired: 10 in]
        n60 = call "雷射_FGV.vi"("Enum"=T10."RS232_Init ", "error in"=w189, "VISA resource name"=w190) -> ()  [unwired: 6 in, 3 out]
      }
      frame "      5.2雷射-寫入數值" {
        n61 = flat-sequence {
          tunnel: [w230] -> w215
          tunnel: ["功率"] -> w212
          tunnel: ["掃描速率(刀速)"] -> w210
          tunnel: ["雷射半徑"] -> w208
          tunnel: ["功率"] -> w207
          tunnel: ["掃描速率(刀速)"] -> w204
          tunnel: w215 -> [w239]
          tunnel: [w239] -> w214
          tunnel: [w237] -> w213
          tunnel: w212 -> [w237]
          tunnel: [w236] -> w211
          tunnel: w210 -> [w236]
          tunnel: [w235] -> w209
          tunnel: w208 -> [w235]
          tunnel: w207 -> [w234]
          tunnel: [w234] -> w206
          tunnel: [w233] -> w205
          tunnel: w204 -> [w233]
          tunnel: w214 -> [w242]
          tunnel: w213 -> [w247]
          tunnel: w211 -> [w246]
          tunnel: w209 -> [w245]
          tunnel: w206 -> [_]
          tunnel: w205 -> [_]
          tunnel: [w247] -> w202
          tunnel: [w246] -> w200
          tunnel: [w245] -> w198
          tunnel: [w243] -> w197
          tunnel: [w241] -> w194
          tunnel: [w252] -> w203
          tunnel: w202 -> [w252]
          tunnel: [w251] -> w201
          tunnel: w200 -> [w251]
          tunnel: [w250] -> w199
          tunnel: w198 -> [w250]
          tunnel: w197 -> [w249]
          tunnel: [w249] -> w196
          tunnel: [w248] -> w195
          tunnel: w194 -> [w248]
          tunnel: w203 -> [w263]
          tunnel: w201 -> [w262]
          tunnel: w199 -> [w261]
          tunnel: w196 -> [w257]
          tunnel: w195 -> [w256]
          frame #0 {
            n62 = call "點檢_雷射_命令(切圓)VI.vi"("半徑"="雷射半徑", "雷射圓心座標"="雷射圓心座標", "掃描速率(刀速)"="掃描速率(刀速)", "功率"="功率") -> ("error out"=w231:errorcluster, "命令字串"=w232:string)  [unwired: 6 in]
            n63 = call "雷射_FGV.vi"("Enum"=T10."寫入雷射XY座標值與角度", "error in"=w231, "命令字串"=w232) -> ("error out"=w230:errorcluster)  [unwired: 6 in, 2 out]
          }
          frame #1 {
            n64 = Wait (ms)(milliseconds to wait=u32 350) -> ()  [unwired: 1 out]
          }
          frame #2 {
            # "將Program值讀出"
            n65 = call "雷射_FGV.vi"("Enum"=T10."寫入雷射XY座標值與角度", "error in"=w242, "命令字串"="F1,0002") -> ("error out"=w241:errorcluster, "回復訊息"=w243:string)  [unwired: 6 in, 1 out]
          }
          frame #3 {
            n66 = Wait (ms)(milliseconds to wait=u32 350) -> ()  [unwired: 1 out]
          }
          frame #4 {
            w268 = "雷射"
            # "將讀出值F1，0及刀數替換"
            n67 = call "RS232_命令(刀數).vi"("error in (no error)"=w256, "program"=enum16{"0000", "0002"}."0002", "刀數"="切割刀數", "回復訊息 3"=w257) -> ("error out"=w260:errorcluster, "result string 3"=w259:string)  [unwired: 6 in]
            n68 = Bundle("功率"=w263, "掃描速率(刀速)"=w262, "雷射半徑"=w261, "切割刀數"="切割刀數") -> (w265:T16)  [unwired: 1 in]
            n69 = To Variant(anything=w265) -> (Variant=w266:variant)
            n70 = call "雷射_FGV.vi"("Enum"=T10."寫入雷射XY座標值與角度", "error in"=w260, "命令字串"=w259) -> ()  [unwired: 6 in, 3 out]
            n71 = Bundle(w268, "Variant"=w266) -> (w267:cluster{string, "Variant":variant})  [unwired: 1 in]
            n72 = call "Main_FGV_Data.vi"("Action_Data"=Action_Data."Set Data", "Data In"=w267, "Data name"=w268) -> ()  [unwired: 7 in, 2 out]
          }
        }
        n73 = disable-structure shown="Disabled" {
          frame Disabled {
            n74 = call "Main_FGV_Data.vi"("Action_Data"=Action_Data."Get Data", "Data name"="參數設定") -> ("Data  Out"=w221:cluster{"Data name":string, "Data":variant})  [unwired: 8 in, 1 out]
            n75 = Unbundle By Name(w221) -> ("Data"=w222:variant)
            n76 = Variant To Data(type=T11 {{"掃描速度"=0, "功率"=0, "切割刀數"=0.0, "左/右"=""}, {"掃描速度2"=0, "功率2"=0, "切割刀數2"=0.0, "左/右"=""}, {"掃描速度3"=0, "功率3"=0, "切割刀數3"=0.0, "左/右"=""}, {"掃描速度4"=0, "功率4"=0, "切割刀數4"=0.0, "左/右"=""}, {"掃描速度5"=0, "功率5"=0, "切割刀數5"=0.0, "左/右"=""}} ("output cluster"), Variant=w222) -> (data=w223:T11)  [unwired: 1 in, 1 out]
            n77 = Unbundle(w223) -> (w218:T17)  [unwired: 4 out]
            n78 = Unbundle By Name(w218) -> ()  [unwired: 4 out]
          }
          frame Enabled {
          }
        }
      }
      frame "      5.3雷射-讀出數值" {
      }
      frame "      5.4雷射-雷射觸發" {
        n79 = flat-sequence {
          tunnel: [w280] -> w271
          tunnel: w271 -> [_]
          frame #0 {
            n80 = Wait (ms)(milliseconds to wait=u32 350) -> ()  [unwired: 1 out]
          }
          frame #1 {
            n81 = call "雷射_FGV.vi"("Enum"=T10."運行切換", "PROGRAM"=enum16{"0000", "0002"}."0002") -> ()  [unwired: 7 in, 3 out]
          }
          frame #2 {
            n82 = Wait (ms)(milliseconds to wait=u32 350) -> ()  [unwired: 1 out]
          }
          frame #3 {
            n83 = call "雷射_FGV.vi"("Enum"=T10."雷射準備訊號") -> ("error out"=w281:errorcluster)  [unwired: 8 in, 2 out]
            n84 = call "雷射_FGV.vi"("Enum"=T10."雷射觸發", "error in"=w281) -> ("error out"=w280:errorcluster)  [unwired: 7 in, 2 out]
          }
          frame #4 {
            n85 = Wait (ms)(milliseconds to wait=u32 850) -> ()  [unwired: 1 out]
          }
        }
      }
      frame "      5.5雷射-關閉" {
        n86 = call "雷射_FGV.vi"("Enum"=T10."RS232_Close") -> ()  [unwired: 8 in, 3 out]
      }
      frame "6.0功能-檔案" {
      }
      frame "       6.1檔案-初始化" {
        n87 = call "Main_FGV_Data.vi"("Action_Data"=Action_Data."Initialize") -> ()  [unwired: 9 in, 2 out]
      }
      frame "       6.2檔案-儲存檔案" {
        w292 = "參數設定" ("name or relative path")
        # "儲存變更參數到參數設定"
        n88 = local read "左/右"() -> (w300:enum16{"オ", "右"})
        n89 = property on="左/右" class="Enum (strict)"() -> ("Strings []"=w302:string[])  [unwired: 2 in, 2 out]
        n90 = To Long Integer(number=w300) -> (32bit integer=w301:i32)
        n91 = Index Array(array=w302, index=w301) -> (element=w297:string)
        n92 = flat-sequence {
          tunnel: w292 -> [w322]
          tunnel: "file (use dialog)" -> [w340]
          tunnel: w292 -> [w339]
          tunnel: [w336] -> _
          frame #0 {
            n93 = local read "掃描速率(刀速)"() -> (w313:u16)
            n94 = local read "切割刀數"() -> (w311:u32)
            n95 = local read "功率"() -> (w305:u8)
            n96 = Unbundle By Name("?") -> ("掃描速度3"=w329:i32, "功率3"=w328:i32, "切割刀數3"=w327:i32, "角度3"=w309:dbl)
            n97 = Unbundle By Name("?") -> ("掃描速度4"=w326:i32, "功率4"=w325:i32, "切割刀數4"=w324:i32, "角度4"=w308:dbl)
            n98 = Unbundle By Name("?") -> ("掃描速度2"=w331:i32, "功率2"=w330:i32, "切割刀數2"=w307:i32, "角度2"=w306:dbl)
            n99 = Unbundle By Name("?") -> ("掃描速度"=w334:i32, "功率"=w333:i32, "切割刀數"=w332:i32, "角度"=w310:dbl)
            n100 = Bundle("掃描速率(刀速)"=w313, "功率"=w305, "切割刀數"=w311) -> (w314:cluster{"掃描速率(刀速) ":u16, "功率":u8, "切割刀數":u32})  [unwired: 1 in]
            n101 = Bundle("掃描速度4"=w326, "功率4"=w325, "切割刀數4"=w324, "角度4"=w308) -> (w318:T18)  [unwired: 1 in]
            n102 = Bundle("掃描速度2"=w331, "功率2"=w330, "切割刀數2"=w307, "角度2"=w306) -> (w320:T19)  [unwired: 1 in]
            n103 = Bundle("掃描速度3"=w329, "功率3"=w328, "切割刀數3"=w327, "角度3"=w309) -> (w319:T20)  [unwired: 1 in]
            n104 = Bundle("掃描速度"=w334, "功率"=w333, "切割刀數"=w332, "角度"=w310) -> (w321:T21)  [unwired: 1 in]
            n105 = Bundle(w321, w320, w319, w318, w314) -> (w317:T1)  [unwired: 1 in]
            "output cluster" <- w317
            n106 = To Variant(anything=w317) -> (Variant=w316:variant)
            n107 = Bundle("name or relative path"=w322, "Variant"=w316) -> (w315:T22)  [unwired: 1 in]
            n108 = call "Main_FGV_Data.vi"("Action_Data"=Action_Data."Set Data", "Data In"=w315, "Data name"=w322) -> ()  [unwired: 7 in, 2 out]
          }
          frame #1 {
            n109 = Build Path(base path=w340, name or relative path=w339) -> (appended path=w337:path)
            n110 = call "Main_FGV_Data.vi"("Action_Data"=Action_Data."Idle") -> ("Data Array out"=w335:cluster{"Data name":string, "Data":variant}[])  [unwired: 9 in, 1 out]
            n111 = Write to Binary File(file (use dialog)=w337, data=w335) -> (error out=w336:errorcluster)  [unwired: 4 in, 2 out]
          }
        }
        n112 = Concatenate Strings("是否要儲存" ("string"), w297, "參數" ("string")) -> (w299:string)
        n113 = Two Button Dialog(message=w299, 1:"否" ("F button name (\"Cancel\")"), 2:"是" ("T button name (\"OK\")")) -> (T button?=w295:bool)
        n114 = case shown="True" w295 {
          tunnel: w297 -> [_ w341]
          frame False {
          }
          frame True {
            n115 = call "Main_FGV_Data.vi"("Action_Data"=Action_Data."Idle") -> ("Data Array out"=w346:cluster{"Data name":string, "Data":variant}[])  [unwired: 9 in, 1 out]
            n116 = Concatenate Strings("點檢Data" ("name or relative path"), w341) -> (w343:string)
            n117 = Build Path(base path=path "C:/Users/noname/Desktop/Main-Page/四穴雷切/Data資料夾/點檢Data" ("file (use dialog) 2"), name or relative path=w343) -> (appended path=w344:path)
            n118 = Write to Binary File(file (use dialog)=w344, data=w346) -> ()  [unwired: 4 in, 3 out]
          }
        }
      }
      frame "       6.3檔案-開啟檔案" {
        n119 = call "File Dialog"("start path"=path "C:/Users/noname/Desktop/Main-Page/四穴雷切/Data資料夾/點檢Data/Data" ("file (use dialog)")) -> ("selected path"=w355:path, "error out"=w349:errorcluster)  [unwired: 11 in, 2 out]
        n120 = call "Main_FGV_Data.vi"("Action_Data"=Action_Data."Initialize") -> ("Data Array out"=w358:cluster{"Data name":string, "Data":variant}[])  [unwired: 9 in, 1 out]
        n121 = Read from Binary File(5:w358, 11:w355) -> (0:w348:errorcluster, 2:w357:cluster{"Data name":string, "Data":variant}[])  [unwired: 4 in, 2 out]
        n122 = for {
          tunnel: w357 -> [w360] mode=indexing
          n123 = Unbundle(w360) -> ("Data name"=w361:string)  [unwired: 1 out]
          n124 = call "Main_FGV_Data.vi"("Action_Data"=Action_Data."Set Data", "Data In"=w360, "Data name"=w361) -> ()  [unwired: 7 in, 2 out]
        }
        n125 = Enqueue Element(queue=w353, element=點檢_Control_Main_Action."       6.4檔案-匯入數值", error in (no error)=w352) -> (queue out=w354:refnum<queue>, error out=w351:errorcluster)  [unwired: 1 in, 1 out]
      }
      frame "       6.4檔案-匯入數值" {
        n126 = local read "左/右"() -> (w381:enum16{"オ", "右"})
        n127 = property on="左/右" class="Enum (strict)"() -> ("Strings []"=w383:string[])  [unwired: 2 in, 2 out]
        n128 = property on="找圓" class="Bool"() -> ("Label.Text"=w380:string)  [unwired: 2 in, 2 out]
        n129 = To Long Integer(number=w381) -> (32bit integer=w382:i32)
        n130 = Index Array(array=w383, index=w382) -> (element=w376:string)
        n131 = Concatenate Strings("Data" ("Data name"), w376) -> (w377:string)
        n132 = Concatenate Strings(w380, w376) -> (w379:string)
        n133 = call "Main_FGV_Data.vi"("Action_Data"=Action_Data."Get Data", "Data name"=w377) -> ("Data  Out"=w393:cluster{"Data name":string, "Data":variant})  [unwired: 8 in, 1 out]
        n134 = call "Main_FGV_Data.vi"("Action_Data"=Action_Data."Get Data", "Data name"=w379) -> ("Data  Out"=w388:cluster{"Data name":string, "Data":variant})  [unwired: 8 in, 1 out]
        n135 = call "Main_FGV_Data.vi"("Action_Data"=Action_Data."Get Data", "Data name"="雷射") -> ("Data  Out"=w371:cluster{"Data name":string, "Data":variant})  [unwired: 8 in, 1 out]
        n136 = Unbundle By Name(w371) -> ("Data"=w370:variant)
        n137 = Unbundle By Name(w393) -> ("Data"=w392:variant)
        n138 = Unbundle By Name(w388) -> ("Data"=w387:variant)
        n139 = Variant To Data(type=T12 {"功率"=0, "掃描速率(刀速) "=0, "雷射半徑"=0.0, "刀數"=0} ("output cluster"), Variant=w370) -> (data=w368:T12, error out=w367:errorcluster)  [unwired: 1 in]
        n140 = Variant To Data(type=cluster{sgl, sgl} {0.0, 0.0} ("x-y"), Variant=w392) -> (data=w390:cluster{sgl, sgl}, error out=w375:errorcluster)  [unwired: 1 in]
        n141 = Variant To Data(type=T13 {"ROI"={"Global Rectangle"=[], "Contours"=[]}, "圓心 (Pixels)"={"X"=0.0, "Y"=0.0}} ("output cluster"), Variant=w387) -> (data=w385:T13, error out=w374:errorcluster)  [unwired: 1 in]
        n142 = Unbundle By Name(w385) -> ("圓心 (Pixels)"=w384:cluster{"X":sgl, "Y":sgl})
        n143 = Unbundle(w368) -> ("功率"=w366:u8, "掃描速率(刀速)"=w365:u16, "雷射半徑"=w364:dbl, "刀數"=w363:u32)
        n144 = local write "原來差值"(w390) -> ()
        n145 = local write "切割刀數"(w363) -> ()
        n146 = local write "功率"(w366) -> ()
        n147 = local write "掃描速率(刀速)"(w365) -> ()
        n148 = local write "雷射半徑"(w364) -> ()
        n149 = local write "原來圓心"(w384) -> ()
      }
      frame "7.0 錯誤" {
      }
      frame "8.0等待" {
      }
      frame "       8.1等待(計算時間)" {
      }
      frame "9.0離開" {
      }
      frame "10.0功能-機台驗證" {
      }
      frame "      10.1機台驗證-測試" {
        n150 = local read "左/右"() -> (w414:enum16{"オ", "右"})
        n151 = property on="左/右" class="Enum (strict)"() -> ("Strings []"=w416:string[])  [unwired: 2 in, 2 out]
        n152 = property on="找圓" class="Bool"() -> ("Label.Text"=w413:string)  [unwired: 2 in, 2 out]
        n153 = To Long Integer(number=w414) -> (32bit integer=w415:i32)
        n154 = Index Array(array=w416, index=w415) -> (element=w410:string)
        n155 = Concatenate Strings(w413, w410) -> (w412:string)
        n156 = call "Main_FGV_Data.vi"("Action_Data"=Action_Data."Get Data", "Data name"=w412) -> ("Data  Out"=w430:cluster{"Data name":string, "Data":variant})  [unwired: 8 in, 1 out]
        n157 = call "Image FGV.vi"("Image action"=Image_action."讀取圖片", "圖片名稱"="Image") -> ("Image Out"=w426:T4)  [unwired: 8 in, 1 out]
        n158 = Unbundle By Name(w430) -> ("Data"=w429:variant)
        n159 = call "IMAQ GetImageSize"("Image"=w426) -> ("Y Resolution"=w432:i32, "X Resolution"=w437:i32)  [unwired: 3 in, 1 out]
        n160 = To Double Precision Float(number=w437) -> (double precision float=w436:dbl)
        n161 = To Double Precision Float(number=w432) -> (double precision float=w433:dbl)
        n162 = Variant To Data(type=T13 {"ROI"={"Global Rectangle"=[], "Contours"=[]}, "圓心 (Pixels)"={"X"=0.0, "Y"=0.0}} ("output cluster"), Variant=w429) -> (data=w427:T13)  [unwired: 1 in, 1 out]
        n163 = Divide(x=w436, y=2.0) -> (x/y=w425:dbl)
        n164 = Divide(x=w433, y=2.0) -> (x/y=w424:dbl)
        n165 = Unbundle(w427) -> ("圓心 (Pixels)"=w417:cluster{"X":sgl, "Y":sgl})  [unwired: 1 out]
        n166 = To Single Precision Float(number=w425) -> (single precision float=w423:sgl)
        n167 = To Single Precision Float(number=w424) -> (single precision float=w422:sgl)
        n168 = Bundle(w423, w422) -> (w418:cluster{sgl, sgl})  [unwired: 1 in]
        n169 = Subtract(x=w417, y=w418) -> (x-y=w420:cluster{sgl, sgl})
        "原來差值" <- w420
        n170 = local write "原來圓心"(w417) -> ()
        n171 = To Variant(anything=w420) -> (Variant=w419:variant)
        n172 = Concatenate Strings("Data" ("Data name"), w410) -> (w409:string)
        n173 = Bundle(w409, "Variant"=w419) -> (w408:cluster{string, "Variant":variant})  [unwired: 1 in]
        n174 = call "Main_FGV_Data.vi"("Action_Data"=Action_Data."Set Data", "Data In"=w408, "Data name"=w409) -> ()  [unwired: 7 in, 2 out]
      }
      frame "      10.2機台驗證-檢測" {
        n175 = property on="Image" class="ImageControl"() -> ("ROI"=w455:T15)  [unwired: 2 in, 2 out]
        n176 = call "Image FGV.vi"("Image action"=Image_action."讀取圖片", "圖片名稱"="Image") -> ("Image Out"=w462:T4)  [unwired: 8 in, 1 out]
        n177 = call "IMAQ GetImageSize"("Image"=w462) -> ("Y Resolution"=w463:i32, "X Resolution"=w468:i32)  [unwired: 3 in, 1 out]
        n178 = call "點檢_VI_找圓.vi"("ROI Descriptor"=w455, "Image"=w462) -> ("圓心 (Pixels)"=w456:cluster{"X":sgl, "Y":sgl})  [unwired: 6 in, 3 out]
        "後來圓心" <- w456
        n179 = To Double Precision Float(number=w468) -> (double precision float=w467:dbl)
        n180 = property on="左/右" class="Enum (strict)"() -> ("Strings []"=w447:string[])  [unwired: 2 in, 2 out]
        n181 = local read "左/右"() -> (w445:enum16{"オ", "右"})
        n182 = To Double Precision Float(number=w463) -> (double precision float=w464:dbl)
        n183 = To Long Integer(number=w445) -> (32bit integer=w446:i32)
        n184 = Divide(x=w467, y=2.0) -> (x/y=w461:dbl)
        n185 = Divide(x=w464, y=2.0) -> (x/y=w460:dbl)
        n186 = Index Array(array=w447, index=w446) -> (element=w442:string)
        n187 = To Single Precision Float(number=w461) -> (single precision float=w459:sgl)
        n188 = To Single Precision Float(number=w460) -> (single precision float=w458:sgl)
        n189 = Bundle(w459, w458) -> (w457:cluster{sgl, sgl})  [unwired: 1 in]
        n190 = Concatenate Strings("Data" ("Data name"), w442) -> (w443:string)
        n191 = Subtract(x=w456, y=w457) -> (x-y=w450:cluster{sgl, sgl})
        "後來差值" <- w450
        n192 = call "Main_FGV_Data.vi"("Action_Data"=Action_Data."Get Data", "Data name"=w443) -> ("Data  Out"=w452:cluster{"Data name":string, "Data":variant})  [unwired: 8 in, 1 out]
        n193 = Unbundle By Name(w452) -> ("Data"=w453:variant)
        n194 = Variant To Data(type=cluster{sgl, sgl} {0.0, 0.0} ("x-y"), Variant=w453) -> (data=w449:cluster{sgl, sgl})  [unwired: 1 in, 1 out]
        n195 = Subtract(x=w450, y=w449) -> (x-y=→"前後差異值":cluster{sgl, sgl})
      }
      frame "11.0對話視窗" {
      }
    }
  }
  n196 = while {
    tunnel: w7 -> [w480]
    tunnel: w6 -> [w479]
    stop <- w478 stop-if-true
    n197 = event shown="[6] \"雷射觸發\": Value Change" {
      selector: _ -> [_ _ _ _ _ _ _ _ _]
      dyn-events: _ -> [_ _ _ _ _ _ _ _ _]
      timeout: _ -> [_ _ _ _ _ _ _ _ _]
      tunnel: w480 -> [w482 w485 w488 w492 w495 w498 w501 w504 w507]
      tunnel: [w482 w485 w488 w492 w495 w498 w501 w504 w507] -> w477
      tunnel: w479 -> [w481 w484 w487 w491 w494 w497 w500 w503 w506]
      tunnel: [w481 w484 w487 w491 w494 w497 w500 w503 w506] -> w476
      tunnel: [_ _ TRUE _ _ _ _ _ _] -> w478
      tunnel: [_ 點檢_Control_Main_Action."二、動作-單次取像" ("element") 點檢_Control_Main_Action."七、動作-離開" ("element") 點檢_Control_Main_Action."      4.2檢測-找圓(原來)" ("element") 點檢_Control_Main_Action."三、動作-測試" ("element") 點檢_Control_Main_Action."四、動作-點檢" ("element") 點檢_Control_Main_Action."六、動作-雷射處發" ("element") 點檢_Control_Main_Action."       6.2檔案-儲存檔案" ("element") 點檢_Control_Main_Action."       6.3檔案-開啟檔案" ("element")] -> w475
      event Timeout {
        n198 = event-data() -> ()  [unwired: 1 in, 3 out]
      }
      event "取像": Value Change {
        n199 = event-data() -> ()  [unwired: 1 in, 1 out]
      }
      event "離開": Value Change {
        n200 = event-data() -> ()  [unwired: 1 in, 1 out]
      }
      event "找圓": Value Change {
        n201 = event-data() -> ()  [unwired: 1 in, 1 out]
      }
      event "差值": Value Change {
        n202 = event-data() -> ()  [unwired: 1 in, 1 out]
      }
      event "點檢": Value Change {
        n203 = event-data() -> ()  [unwired: 1 in, 1 out]
      }
      event "雷射觸發": Value Change {
        n204 = event-data() -> ()  [unwired: 1 in, 1 out]
      }
      event "儲存檔案": Value Change {
        n205 = event-data() -> ()  [unwired: 1 in, 1 out]
      }
      event "開啟檔案": Value Change {
        n206 = event-data() -> ()  [unwired: 1 in, 1 out]
      }
    }
    n207 = Enqueue Element(queue=w477, element=w475, error in (no error)=w476) -> ()  [unwired: 1 in, 3 out]
  }
  n208 = Release Queue(queue=w5, error in (no error)=w4) -> ()  [unwired: 1 in, 3 out]
